vi "sub_udp_item-sel.vi"(7 "item":T3=enum."ip", 11 "get-data":string) -> (0 "dbl":dbl, 1 "watchdogval":i32, 2 "Error Display":T2={"AGV"=2, "AGV Estop"=0, "Obstacle"=1, "GNSS"=2, "TIM571"=2, "Cam"=2, "Joystick"=1}, 3 "out":string)   [LabVIEW 2019]
uses:
  Ctrl/udp_item.ctl
  Ctrl/status.ctl
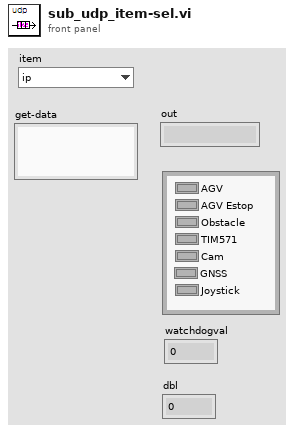
[diagram p1: front panel]
types:
  T1 = typedef "status.ctl" = u16
  T2 = cluster{"AGV":T1, "AGV Estop":T1, "Obstacle":T1, "GNSS":T1, "TIM571":T1, "Cam":T1, "Joystick":T1}
  T3 = typedef "udp_item.ctl" = enum16{"Long", "Lat", "watchdog", "Scoutmini", "RBAstatus", "Err", "ip", "VLp", "VAp", "Batt"}
  T4 = cluster{"배열 타입(2D Dbl)[0]":u8, "배열 타입(2D Dbl)[1]":u8, "배열 타입(2D Dbl)[2]":u8, "배열 타입(2D Dbl)[3]":u8, "배열 타입(2D Dbl)[4]":u8, "배열 타입(2D Dbl)[5]":u8, "배열 타입(2D Dbl)[6]":u8}
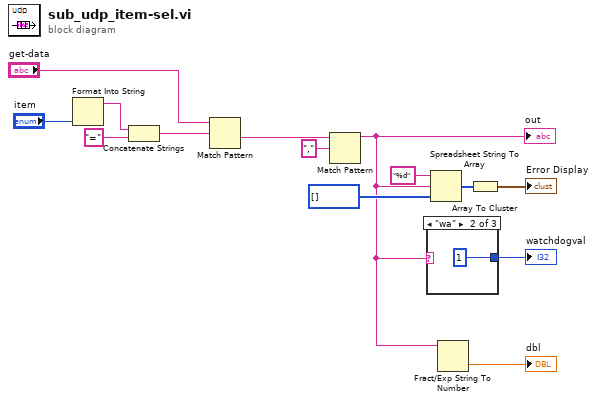
[diagram p0: block diagram]
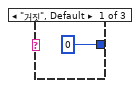
[diagram p2: hidden frame]
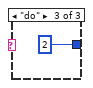
[diagram p3: hidden frame]
diagram:
  n1 = Format Into String("item") -> (resulting string=w9:string)  [unwired: 3 in, 1 out]
  n2 = Concatenate Strings(w9, "=" ("문자열")) -> (w11:string)
  n3 = Match Pattern(string="get-data", regular expression=w11) -> (after substring=w3:string)  [unwired: 1 in, 3 out]
  n4 = Match Pattern(string=w3, regular expression="," ("문자열")) -> (before substring=w2:string)  [unwired: 1 in, 3 out]
  "out" <- w2
  n5 = case shown="\"wa\"" w2 {
    tunnel: [0 1 2] -> w4
    frame "거짓", Default {
    }
    frame "wa" {
    }
    frame "do" {
    }
  }
  "watchdogval" <- w4
  n6 = Spreadsheet String To Array(format string="%d" ("포맷 문자열"), spreadsheet string=w2, array type (2D Dbl)=u8[] [] ("배열 타입(2D Dbl)")) -> (array=w12:u8[])  [unwired: 1 in]
  n7 = Fract/Exp String To Number(string=w2) -> (number=→"dbl":dbl)  [unwired: 3 in, 1 out]
  n8 = Array To Cluster(array=w12) -> (cluster=→"Error Display":T4)
